vi "Update sim globals from JSON protocol.vi"(10 "Initialize":bool, 11 "Data":string) -> (1 "SimDevice":bool)   [LabVIEW 2019]
uses:
  <vilib>/MultiError/TokenizeJSON/Multi Error Cluster.lvlib
  Devices/RoboRIO/RoboRIO Update Ops.ctl
  Devices/Relay/Relay Update Ops.ctl
  Devices/PWM/PWM Update Ops.ctl
  Devices/Joystick/Joystick Update Ops.ctl
  Devices/Gyro/Gyro Update Ops.ctl
  Devices/Encoder/Encoder Update Ops.ctl
  Devices/DutyCycle/DutyCycle Update Ops.ctl
  Devices/DriverStation/DS Update Ops.ctl
  Devices/dPWM/dPWM Update Ops.ctl
  Devices/DIO/DIO Update Ops.ctl
  Devices/AO/AO Update Ops.ctl
  Devices/AI/AI Update Ops.ctl
  Devices/Accel/Accel Update Ops.ctl
  Devices/CTREPCM/CTREPCM Update Ops.ctl
  Devices/Solenoid/Solenoid Update Ops.ctl
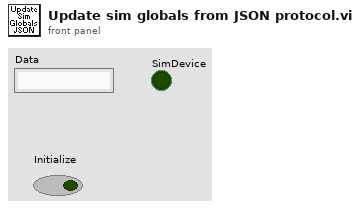
[diagram p1: front panel]
types:
  T1 = cluster{string[], refnum<vi>[], cluster{"index of element":i32, "index of element":i32}[]}
  T2 = typedef "Multi Error Cluster.lvlib/JSON Token Descriptor.ctl" = cluster{"match string":string, "raw token type":T3, "byte offset ":i32}
  T3 = typedef "Multi Error Cluster.lvlib/JSON Raw Token Values.ctl" = enum32{"{", "}", "[", "]", ",", ":", "\"", "number", "string", "true", "false", "null", "invalid"}
  T4 = typedef "Multi Error Cluster.lvlib/JSON Token Values.ctl" = enum32{"array begin", "array end", "object begin", "object end", "value", "invalid", "name"}
  T5 = cluster{"whole match":string, "token index":i32}[]
  T6 = typedef "Accel Update Ops.ctl" = enum16{"get", "delete", "JSON update", "set  name", "transmit initial", "reset", "set init", "set range"}
  T7 = typedef "AI Update Ops.ctl" = enum16{"set init", "set avg_bits", "set oversample_bits", "set voltage", "set Accum_init", "set Accum_value", "set Accum_count", "set Accum_center", "set Accum_deadband", "get", "delete", "JSON update", "set  name", "transmit initial", "reset"}
  T8 = typedef "AO Update Ops.ctl" = enum16{"set init", "set value", "JSON update", "set name", "transmit initial", "get", "delete", "reset"}
  T9 = typedef "DIO Update Ops.ctl" = enum16{"set init", "set value", "set pulse_length", "set input", "get", "delete", "JSON update", "set name", "transmit initial", "reset"}
  T10 = typedef "dPWM Update Ops.ctl" = enum16{"get", "delete", "JSON update", "set  name", "transmit initial", "reset", "set init", "set duty cycle", "set dio channel"}
  T11 = typedef "DS Update Ops.ctl" = enum16{"set enabled", "set autonomous", "set test", "set estop", "set fms", "set ds", "set control word", "set match_time", "set station", "set game data", "JSON update", "set name", "get", "transmit initial", "reset"}
  T12 = typedef "DutyCycle Update Ops.ctl" = enum16{"get", "delete", "JSON update", "set  name", "transmit initial", "reset", "set init"}
  T13 = typedef "Encoder Update Ops.ctl" = enum16{"set init", "set count", "set period", "set reset", "set samples_to_avg", "get", "delete", "JSON update", "set name", "transmit initial", "reset", "set channel_a", "set channel_b"}
  T14 = typedef "Gyro Update Ops.ctl" = enum16{"get", "delete", "JSON update", "set  name", "transmit initial", "reset", "set init", "set offsetX", "set offsetY", "set offsetZ", "set gain", "set angle X", "set angle Y", "set angle Z", "set rate X", "set rate Y", "set rate Z"}
  T15 = typedef "Joystick Update Ops.ctl" = enum16{"set init", "set buttons", "set povs", "set axes", "set left_rumble", "set right_rumble", "set outputs", "get", "delete", "JSON update", "set name", "transmit initial", "reset"}
  T16 = typedef "PWM Update Ops.ctl" = enum16{"set init", "set speed", "set position", "set raw", "set  period_scale", "set zero_latch", "set angular range", "get", "delete", "JSON update", "set name", "transmit initial", "reset"}
  T17 = typedef "Relay Update Ops.ctl" = enum16{"set init_fwd", "set init_rev", "set fwd", "set rev", "get", "delete", "JSON update", "set name", "transmit initial", "reset"}
  T18 = typedef "RoboRIO Update Ops.ctl" = enum16{"get", "JSON update", "set name", "transmit initial", "set fpga_button", "set vin_voltage", "set vin_current", "set 6v_voltage", "set 6v_current", "set 6v_active", "set 6v_faults", "set 5v_voltage", "set 5v_current", "set 5v_active", "set 5v_faults", "set 3v3_voltage", "set 3v3_current", "set 3v3_active", "set 3v3_faults", "reset"}
  T19 = typedef "CTREPCM Update Ops.ctl" = enum16{"get", "delete", "JSON update", "set  name", "transmit initial", "reset", "set init", "set compressor on", "set closed loop", "set pressure switch", "set current"}
  T20 = typedef "Solenoid Update Ops.ctl" = enum16{"get", "delete", "JSON update", "set  name", "transmit initial", "reset", "set init", "set output"}
  T21 = cluster{"index of element":i32, "index of element":i32}[]
  T22 = cluster{"index of element":i32, "index of element":i32}
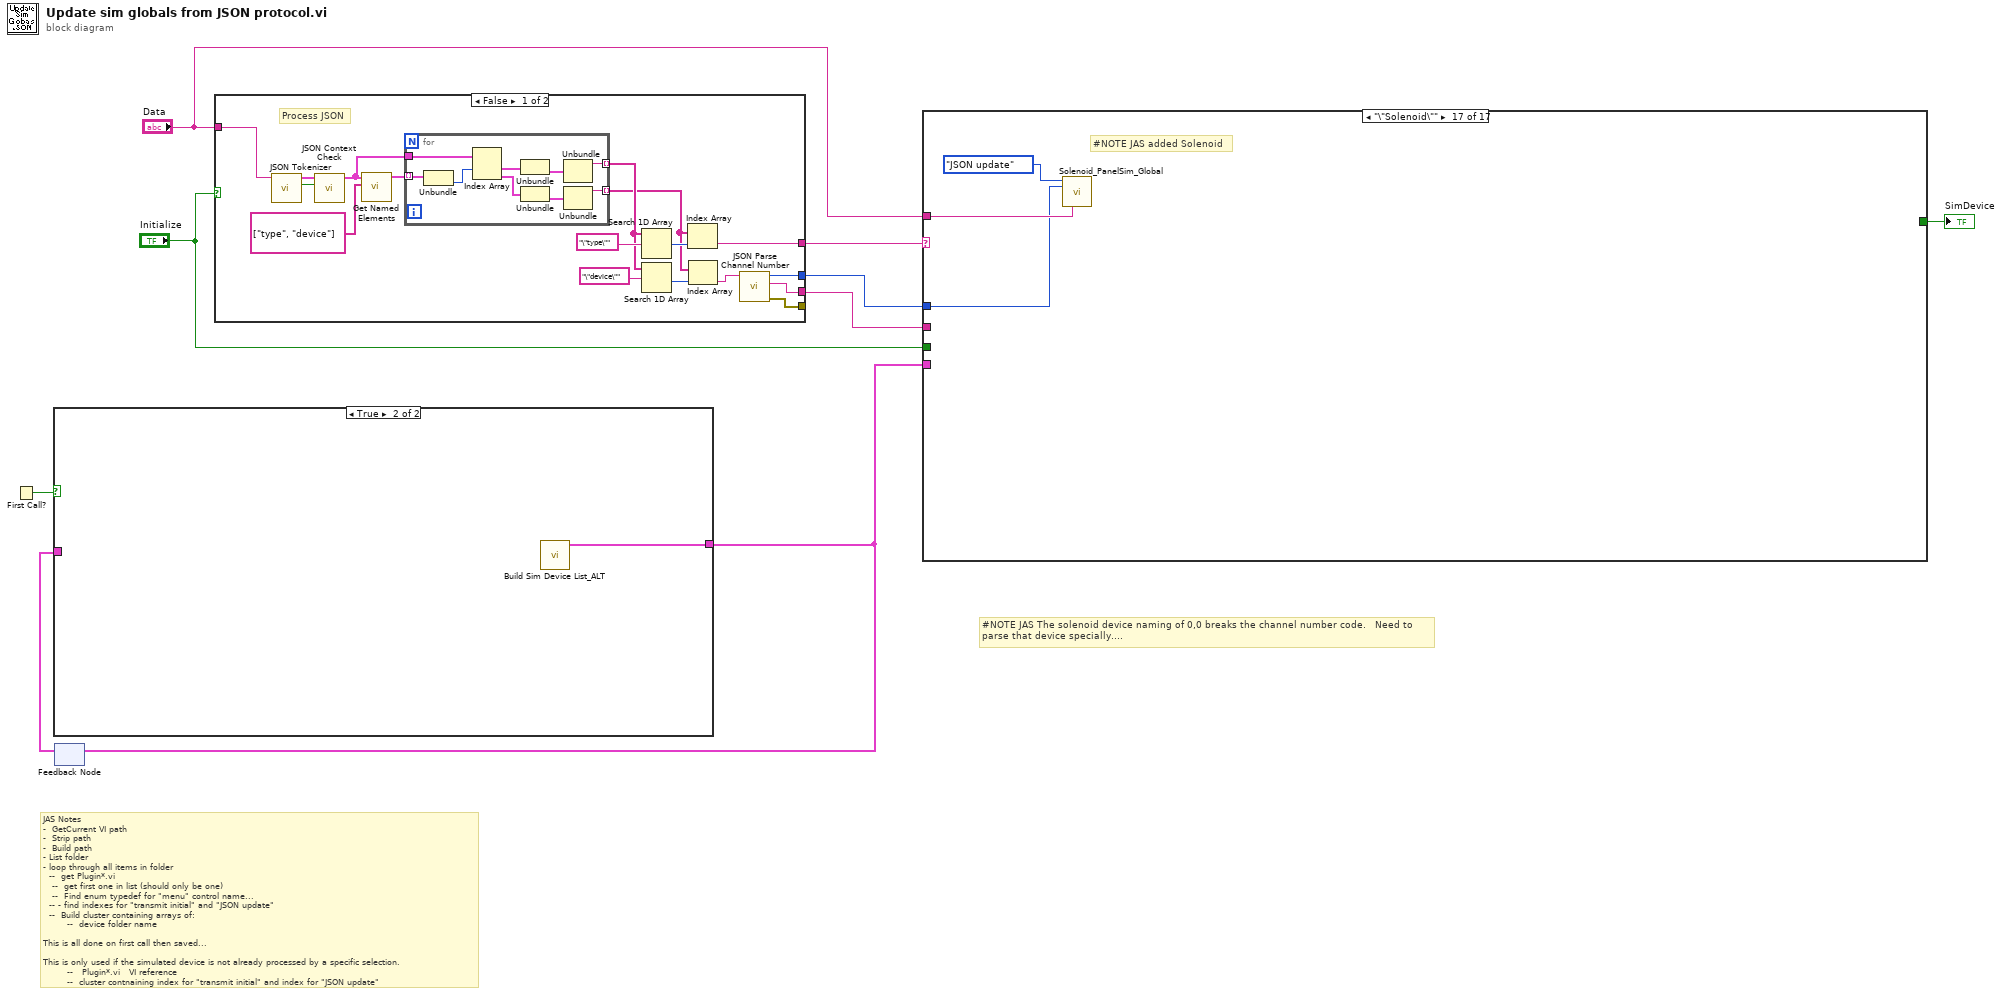
[diagram p0: block diagram]
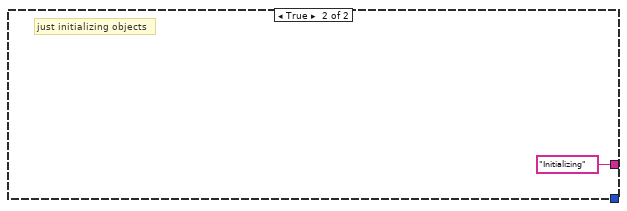
[diagram p2: hidden frame]
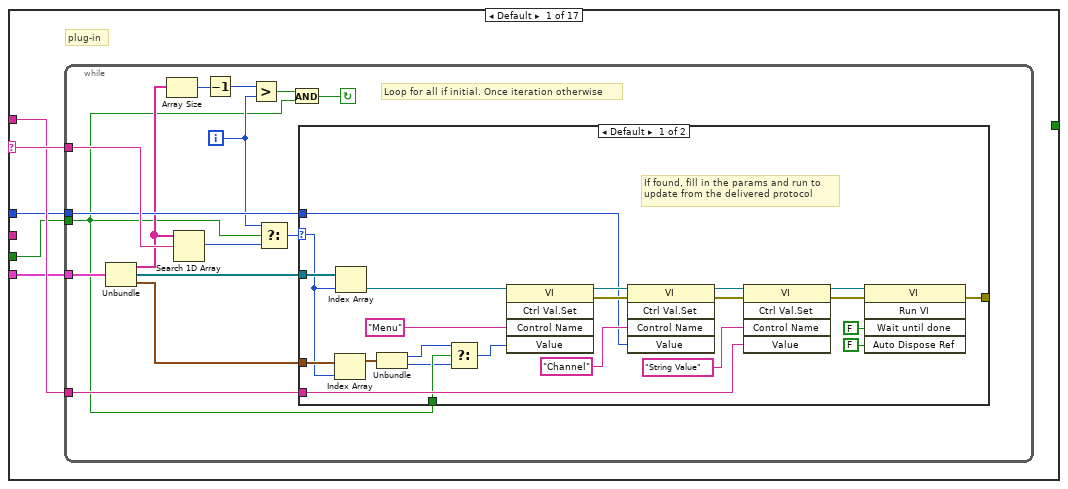
[diagram p4: hidden frame]
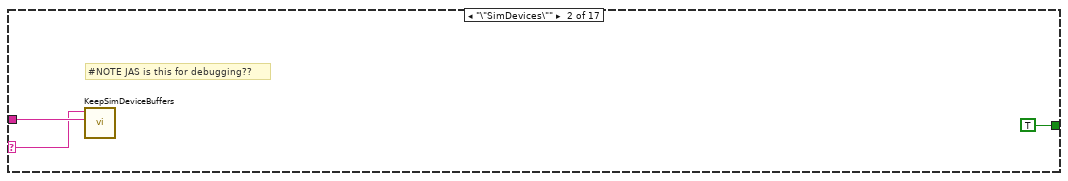
[diagram p6: hidden frame]
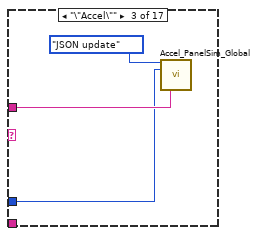
[diagram p7: hidden frame]
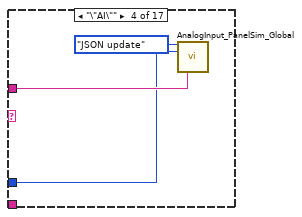
[diagram p8: hidden frame]
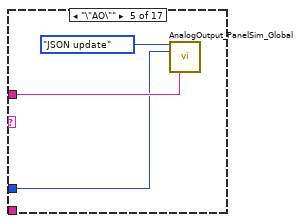
[diagram p9: hidden frame]
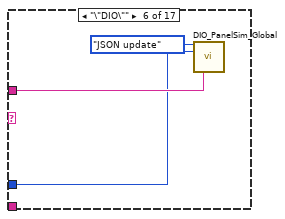
[diagram p10: hidden frame]
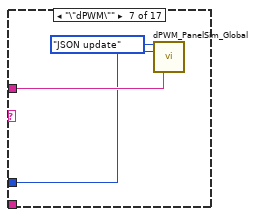
[diagram p11: hidden frame]
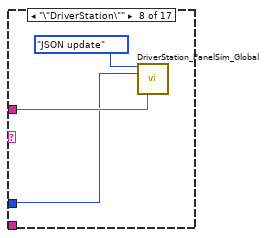
[diagram p12: hidden frame]
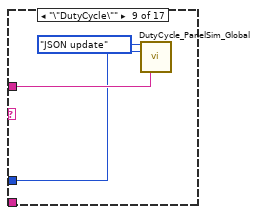
[diagram p13: hidden frame]
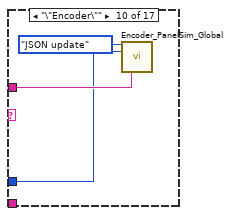
[diagram p14: hidden frame]
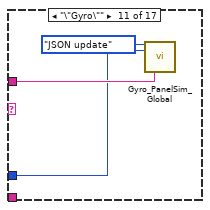
[diagram p15: hidden frame]
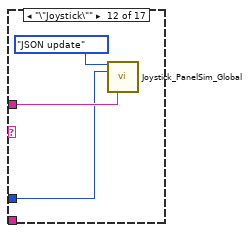
[diagram p16: hidden frame]
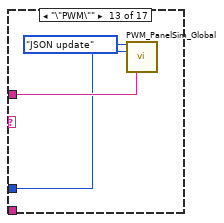
[diagram p17: hidden frame]
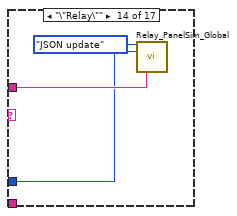
[diagram p18: hidden frame]
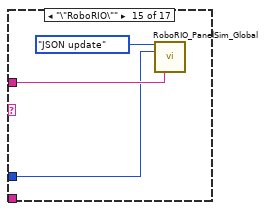
[diagram p19: hidden frame]
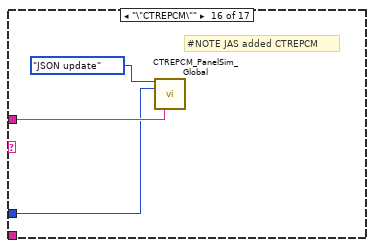
[diagram p20: hidden frame]
diagram:
  # "JAS Notes\n-  GetCurrent VI path\n-  Strip path\n-  Build path\n- List folder\n- loop through all items in folder\n  --  get Plugin*.vi\n   --  get first one in list (should only be one)\n   --  Find enum typedef for \"menu\" control name... \n  -- - find indexes for \"transmit initial\" and \"JSON update\"\n  --  Build cluster containing arrays of:\n        --  device folder name\n\nThis is all done on first call then saved...\n\nThis is only used if the simulated device is not already processed by a specific selection.\n        --   Plugin*.vi   VI reference\n        --  cluster contnaining index for \"transmit initial\" and index for \"JSON update\""
  # "#NOTE JAS The solenoid device naming of 0,0 breaks the channel number code.   Need to\nparse that device specially...."
  n1 = First Call?() -> (First Call?: T/F=w6:bool)
  n2 = feedback #1() -> (w5:T1)  [unwired: 1 in]
  n3 = case shown="True" w6 {
    tunnel: [w10 w11] -> w3
    tunnel: w5 -> [w10 _]
    frame False {
    }
    frame True {
      n4 = call "Build Sim Device List_ALT.vi"() -> ("Sim Device List"=w11:T1)  [unwired: 11 in]
    }
  }
  n5 = feedback-in #1(w3) -> ()
  n6 = case shown="False" "Initialize" {
    tunnel: [w28 "Initializing" ("whole match")] -> w9
    tunnel: "Data" -> [w27 _]
    tunnel: [w14 _] -> w8
    tunnel: [w13 _] -> _
    tunnel: [w12 _] -> w1
    frame False {
      # "Process JSON"
      n7 = call <vilib>:"JSON Tokenizer.vi"("JSON String"=w27) -> ("Invalid"=w21:bool, "Array"=w20:T2[])  [unwired: 9 in]
      n8 = call <vilib>:"JSON Context Check.vi"("Invalid in"=w21, "Parse Tokens in"=w20) -> ("tokens"=w25:cluster{"token type":T4, T2}[])  [unwired: 8 in, 1 out]
      n9 = call <vilib>:"Get Named Elements.vi"("names"=string[] ["type", "device"], "tokens"=w25) -> ("Found Token Info"=w22:T5)  [unwired: 9 in]
      n10 = for {
        tunnel: w22 -> [w37] mode=indexing
        tunnel: w25 -> [w36]
        tunnel: [w32] -> w18 mode=indexing
        tunnel: [w29] -> w17 mode=indexing
        n11 = Unbundle(w37) -> ("token index"=w35:i32)  [unwired: 1 out]
        n12 = Index Array(array=w36, index #1=w35) -> (element #1=w34:cluster{"token type":T4, T2}, element #2=w30:cluster{"token type":T4, T2})  [unwired: 1 in]
        n13 = Unbundle(w34) -> (w33:T2)  [unwired: 1 out]
        n14 = Unbundle(w30) -> (w31:T2)  [unwired: 1 out]
        n15 = Unbundle(w33) -> ("match string"=w32:string)  [unwired: 2 out]
        n16 = Unbundle(w31) -> ("match string"=w29:string)  [unwired: 2 out]
      }
      n17 = Search 1D Array(1D array=w18, element="\"type\"" ("whole match")) -> (index of element=w24:i32)  [unwired: 1 in]
      n18 = Search 1D Array(1D array=w18, element="\"device\"" ("whole match")) -> (index of element=w16:i32)  [unwired: 1 in]
      n19 = Index Array(array=w17, index=w24) -> (element=w28:string)
      n20 = Index Array(array=w17, index=w16) -> (element=w15:string)
      n21 = call "JSON Parse Channel Number.vi"("device string"=w15) -> ("error out"=w13:errorcluster, "Device Subtype"=w12:string, "Channel"=w14:i32)  [unwired: 8 in]
    }
    frame True {
      # "just initializing objects"
    }
  }
  n22 = case shown="\"\\\"Solenoid\\\"\"" w9 {
    selector: w9 -> [w43 w83 _ _ _ _ _ _ _ _ _ _ _ _ _ _ _]
    tunnel: "Data" -> [w42 w84 w87 w90 w93 w96 w99 w102 w105 w108 w111 w114 w117 w120 w123 w126 w129]
    tunnel: w8 -> [w41 _ w85 w88 w92 w95 w98 w100 w104 w107 w110 w112 w116 w119 w122 w125 w128]
    tunnel: [_ TRUE _ _ _ _ _ _ _ _ _ _ _ _ _ _ _] -> w7
    tunnel: w3 -> [w40 _ _ _ _ _ _ _ _ _ _ _ _ _ _ _ _]
    tunnel: "Initialize" -> [w39 _ _ _ _ _ _ _ _ _ _ _ _ _ _ _ _]
    tunnel: w1 -> [_ _ _ _ _ _ _ _ _ _ _ _ _ _ _ _ _]
    frame Default {
      # "plug-in"
      n23 = while {
        tunnel: w43 -> [w58]
        tunnel: w42 -> [w57]
        tunnel: w41 -> [w56]
        tunnel: w40 -> [w55]
        tunnel: w39 -> [w44]
        i -> [w48]
        stop <- w45 continue-if-true
        # "Loop for all if initial. Once iteration otherwise"
        n24 = Unbundle(w55) -> (w50:string[], w54:refnum<vi>[], w51:T21)
        n25 = Array Size(array=w50) -> (size(s)=w49:i32)
        n26 = Search 1D Array(1D array=w50, element=w58) -> (index of element=w52:i32)  [unwired: 1 in]
        n27 = Decrement(x=w49) -> (x-1=w47:i32)
        n28 = Greater?(x=w47, y=w48) -> (0:w46:bool)
        n29 = Select(t=w48, s=w44, f=w52) -> (s? t:f=w53:i32)
        n30 = And(x=w46, y=w44) -> (x .and. y?=w45:bool)
        n31 = case shown="Default" w53 {
          selector: w53 -> [w65 _]
          tunnel: w54 -> [w81 _]
          tunnel: w57 -> [w75 _]
          tunnel: [w69 _] -> _
          tunnel: w51 -> [w66 _]
          tunnel: w44 -> [w63 _]
          tunnel: w56 -> [w59 _]
          frame Default {
            # "If found, fill in the params and run to\nupdate from the delivered protocol"
            n32 = Index Array(array=w66, index=w65) -> (element=w64:T22)
            n33 = Index Array(array=w81, index=w65) -> (element=w68:refnum<vi>)
            n34 = Unbundle(w64) -> ("index of element"=w62:i32, "index of element"=w61:i32)
            n35 = Select(t=w62, s=w63, f=w61) -> (s? t:f=w60:i32)
            n36 = invoke class="VI" method="Ctrl Val.Set"(reference=w68, "Control Name"="Menu" ("whole match"), "Value"=w60) -> (reference out=w80:refnum<vi>, error out=w72:errorcluster)  [unwired: 2 in, 3 out]
            n37 = invoke class="VI" method="Ctrl Val.Set"(reference=w80, error in=w72, "Control Name"="Channel" ("whole match"), "Value"=w59) -> (reference out=w79:refnum<vi>, error out=w71:errorcluster)  [unwired: 1 in, 3 out]
            n38 = invoke class="VI" method="Ctrl Val.Set"(reference=w79, error in=w71, "Control Name"="String Value" ("whole match"), "Value"=w75) -> (reference out=w78:refnum<vi>, error out=w70:errorcluster)  [unwired: 1 in, 3 out]
            n39 = invoke class="VI" method="Run VI"(reference=w78, error in=w70, "Wait until done"=FALSE ("Wait Until Done"), "Auto Dispose Ref"=FALSE ("Auto Dispose Reference")) -> (error out=w69:errorcluster)  [unwired: 1 in, 4 out]
          }
          frame -1 {
            # "not found"
          }
        }
      }
    }
    frame "\"SimDevices\"" {
      # "#NOTE JAS is this for debugging??"
      n40 = call <vilib>:"KeepSimDeviceBuffers.vi"("Bufer"=w84, "Type of device"=w83) -> ()  [unwired: 10 in]
    }
    frame "\"Accel\"" {
      n41 = call "Accel_PanelSim_Global.vi"("Menu"=Accel_Update_Ops."JSON update", "Channel"=w85, "String Value"=w87) -> ()  [unwired: 11 in, 2 out]
    }
    frame "\"AI\"" {
      n42 = call "AnalogInput_PanelSim_Global.vi"("menu"=AI_Update_Ops."JSON update", "Channel"=w88, "String Value"=w90) -> ()  [unwired: 11 in, 2 out]
    }
    frame "\"AO\"" {
      n43 = call "AnalogOutput_PanelSim_Global.vi"("menu"=AO_Update_Ops."JSON update", "AO Channel"=w92, "JSON"=w93) -> ()  [unwired: 11 in, 2 out]
    }
    frame "\"DIO\"" {
      n44 = call "DIO_PanelSim_Global.vi"("menu"=DIO_Update_Ops."JSON update", "DIO Channel"=w95, "String Value"=w96) -> ()  [unwired: 11 in, 2 out]
    }
    frame "\"dPWM\"" {
      n45 = call "dPWM_PanelSim_Global.vi"("Menu"=dPWM_Update_Ops."JSON update", "DIO Channel"=w98, "String Value"=w99) -> ()  [unwired: 11 in, 2 out]
    }
    frame "\"DriverStation\"" {
      n46 = call "DriverStation_PanelSim_Global.vi"("menu"=DS_Update_Ops."JSON update", "Channel"=w100, "String Value"=w102) -> ()  [unwired: 11 in, 2 out]
    }
    frame "\"DutyCycle\"" {
      n47 = call "DutyCycle_PanelSim_Global.vi"("Menu"=DutyCycle_Update_Ops."JSON update", "Channel"=w104, "String Value"=w105) -> ()  [unwired: 11 in, 2 out]
    }
    frame "\"Encoder\"" {
      n48 = call "Encoder_PanelSim_Global.vi"("menu"=Encoder_Update_Ops."JSON update", "EncoderIndex"=w107, "String Value"=w108) -> ()  [unwired: 11 in, 2 out]
    }
    frame "\"Gyro\"" {
      n49 = call "Gyro_PanelSim_Global.vi"("Menu"=Gyro_Update_Ops."JSON update", "Channel"=w110, "String Value"=w111) -> ()  [unwired: 11 in, 2 out]
    }
    frame "\"Joystick\"" {
      n50 = call "Joystick_PanelSim_Global.vi"("menu"=Joystick_Update_Ops."JSON update", "JoystickDevice"=w112, "String Value"=w114) -> ()  [unwired: 11 in, 2 out]
    }
    frame "\"PWM\"" {
      n51 = call "PWM_PanelSim_Global.vi"("menu"=PWM_Update_Ops."JSON update", "PWMChannel"=w116, "String Value"=w117) -> ()  [unwired: 11 in, 2 out]
    }
    frame "\"Relay\"" {
      n52 = call "Relay_PanelSim_Global.vi"("menu"=Relay_Update_Ops."JSON update", "RelayChannel"=w119, "String Value"=w120) -> ()  [unwired: 11 in, 2 out]
    }
    frame "\"RoboRIO\"" {
      n53 = call "RoboRIO_PanelSim_Global.vi"("Menu"=RoboRIO_Update_Ops."JSON update", "Channel"=w122, "String Value"=w123) -> ()  [unwired: 11 in, 2 out]
    }
    frame "\"CTREPCM\"" {
      # "#NOTE JAS added CTREPCM"
      n54 = call "CTREPCM_PanelSim_Global.vi"("Menu"=CTREPCM_Update_Ops."JSON update", "Channel"=w125, "String Value"=w126) -> ()  [unwired: 11 in, 2 out]
    }
    frame "\"Solenoid\"" {
      # "#NOTE JAS added Solenoid"
      n55 = call "Solenoid_PanelSim_Global.vi"("Menu"=Solenoid_Update_Ops."JSON update", "Channel"=w128, "String Value"=w129) -> ()  [unwired: 11 in, 2 out]
    }
  }
  "SimDevice" <- w7
